vi "Display Emoji.vi"(8 "error in (no error)":errorcluster, 10 "Emoji":T1 items=["smile", "laugh", "sad", "mad", "angry", "cry", "greedy", "cool", "shy", "awkward", "heart", "small heart", "broken heart", "waterdrop", "flame", "creeper", "mad creeper", "sword", "wooden sword", "crystal sword", "house", "tree", "flower", "umbrella", "rain", "monster", "crab", "duck", "rabbit", "cat", "up", "down", "left", "right", "smiley face"], 11 "Grove 2 RGB LED Matrix In":refnum<class "Grove 2 RGB LED Matrix.lvclass">) -> (0 "error out":errorcluster, 3 "Grove 2 RGB LED Matrix Out":refnum<class "Grove 2 RGB LED Matrix.lvclass">)   [LabVIEW 2020, in "CTI-Peripheral.lvlib" / "Grove 2 RGB LED Matrix.lvclass"]
uses:
  Grove 2 RGB LED Matrix.lvclass
  Data Types/Emojis.ctl
  Data Types/MatrixI2CCommand.ctl
  Grove 2 RGB LED Matrix.lvclass/Grove 2 RGB LED Matrix.ctl
  CTI/I2C Connection/I2C Connection.lvclass/I2C Connection.ctl
  CTI/Session/I2C Write Data.vi
  CTI/I2C Connection/I2C Connection.lvclass
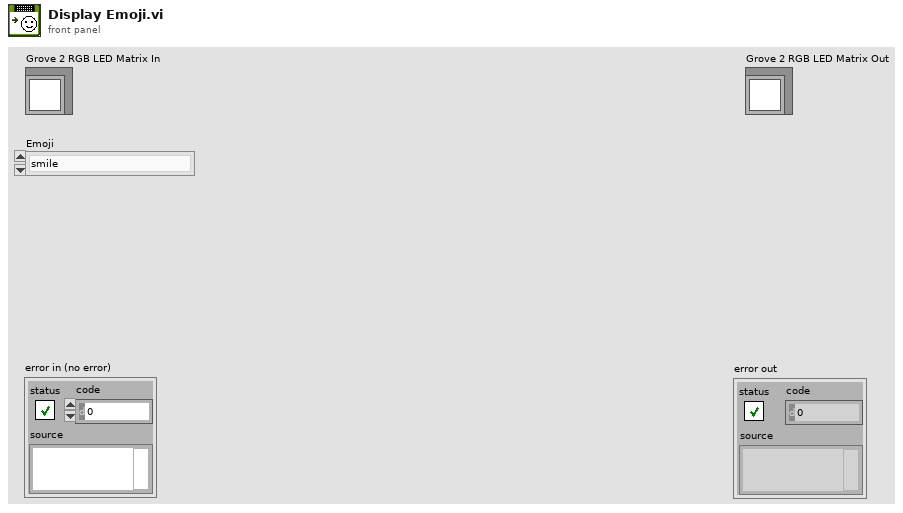
[diagram p1: front panel]
types:
  T1 = typedef "Emojis.ctl" = u16
  T2 = typedef "CTI-Peripheral.lvlib/Grove 2 RGB LED Matrix.lvclass/MatrixI2CCommand.ctl" = u8
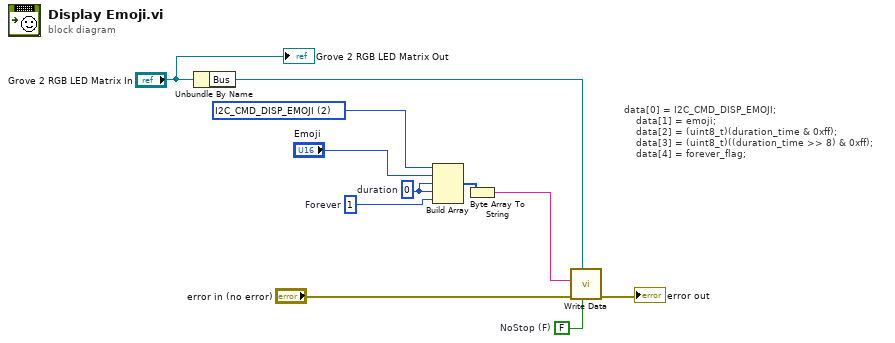
[diagram p0: block diagram]
diagram:
  w2 = u8 0  # duration
  w8 = FALSE  # NoStop (F)
  w1 = u8 1  # Forever
  w9 = T2 2 items=["I2C_CMD_GET_DEV_ID"=0, "I2C_CMD_DISP_BAR"=1, "I2C_CMD_DISP_EMOJI"=2, "I2C_CMD_DISP_NUM"=3, "I2C_CMD_DISP_STR"=4, "I2C_CMD_DISP_CUSTOM"=5, "I2C_CMD_DISP_OFF"=6, "I2C_CMD_DISP_ASCII"=7, "I2C_CMD_DISP_FLASH"=8, "I2C_CMD_DISP_COLOR_BAR"=9, "I2C_CMD_DISP_COLOR_WAVE"=10, "I2C_CMD_DISP_COLOR_CLOCKWISE"=11, "I2C_CMD_DISP_COLOR_ANIMATION"=12, "I2C_CMD_DISP_COLOR_BLOCK "=13, "I2C_CMD_STORE_FLASH"=160, "I2C_CMD_DELETE_FLASH"=161, "I2C_CMD_LED_ON"=176, "I2C_CMD_LED_OFF"=177, "I2C_CMD_AUTO_SLEEP_ON"=178, "I2C_CMD_AUTO_SLEEP_OFF"=179, "I2C_CMD_DISP_ROTATE"=180, "I2C_CMD_DISP_OFFSET"=181, "I2C_CMD_SET_ADDR"=192, "I2C_CMD_RST_ADDR"=193, "I2C_CMD_TEST_GET_VER"=226, "I2C_CMD_GET_DEVICE_UID"=241] ("I2C Command")
  # "data[0] = I2C_CMD_DISP_EMOJI;\n    data[1] = emoji;\n    data[2] = (uint8_t)(duration_time & 0xff);\n    data[3] = (uint8_t)((duration_time >> 8) & 0xff);\n    data[4] = forever_flag;"
  n1 = Unbundle By Name("Grove 2 RGB LED Matrix In") -> ("Bus"=w6:refnum<class "I2C Connection.lvclass">)
  n2 = Build Array(w9, "Emoji", w2, w2, w1) -> (w10:T1[])
  n3 = Byte Array To String(unsigned byte array=w10) -> (string=w5:string)
  n4 = call "Write Data.vi"("NoStop (F)"=w8, "I2C Connection"=w6, "error in (no error)"="error in (no error)", "Data"=w5) -> ("error out"=→"error out":errorcluster)  [unwired: 7 in]
  "Grove 2 RGB LED Matrix Out" <- "Grove 2 RGB LED Matrix In"
